vi "getStatusTime.vi"(0 "String":string, 5 "Time":dbl format="%.2f", 9 "Site":i32) -> (2 "Run":i32, 3 "RunP":i32, 4 "Down":i32, 6 "Repair":i32, 8 "Setup":i32, 10 "SetupW":i32, 13 "PM":i32, 14 "Eng":i32, 15 "Idle":i32)   [LabVIEW 2012]
panel:
  out "Repair":string
  out "PM":string
  out "Eng":string
  out "SetupW":string
  out "Setup":string
  out "Idle":string
  out "Run":string
  out "RunP":string
  out "Down":string
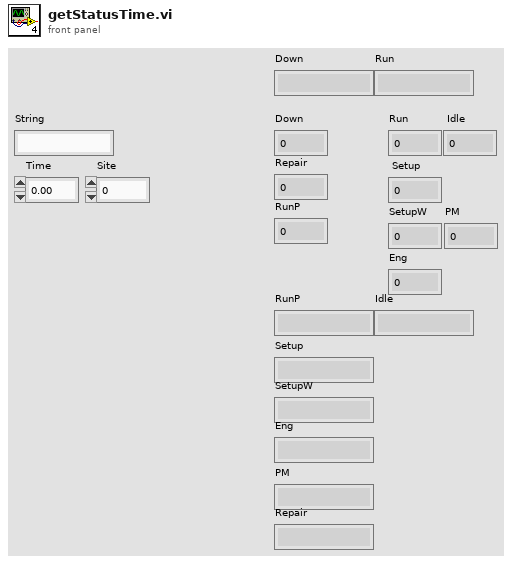
[diagram p1: front panel]
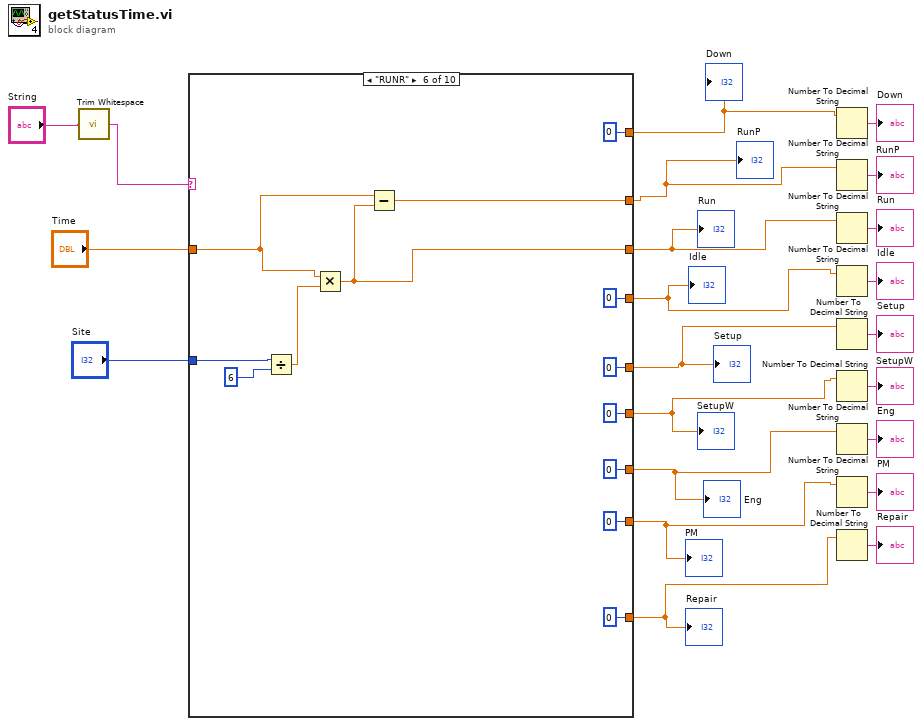
[diagram p0: block diagram]
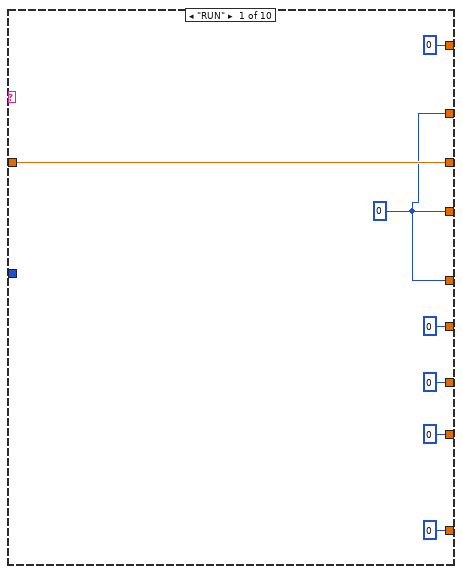
[diagram p2: hidden frame]
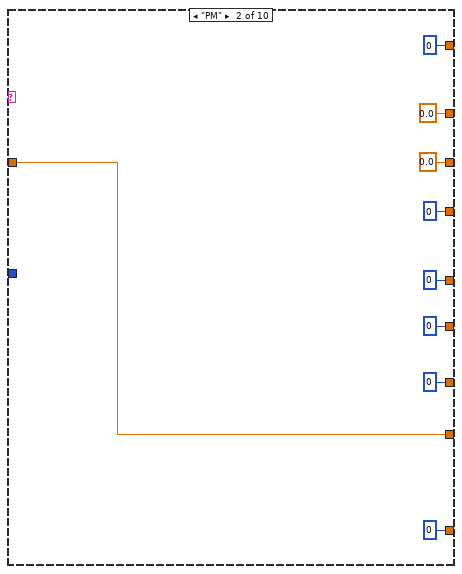
[diagram p3: hidden frame]
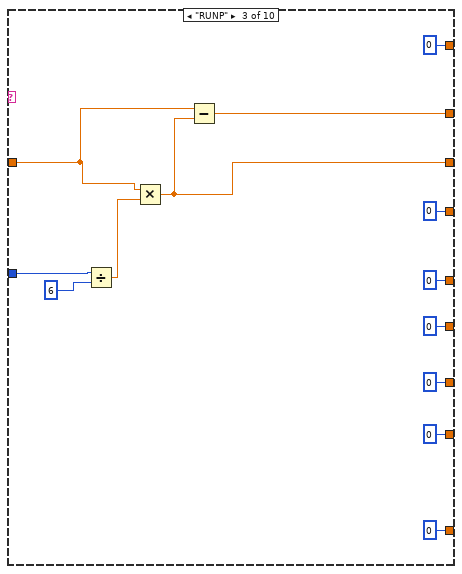
[diagram p4: hidden frame]
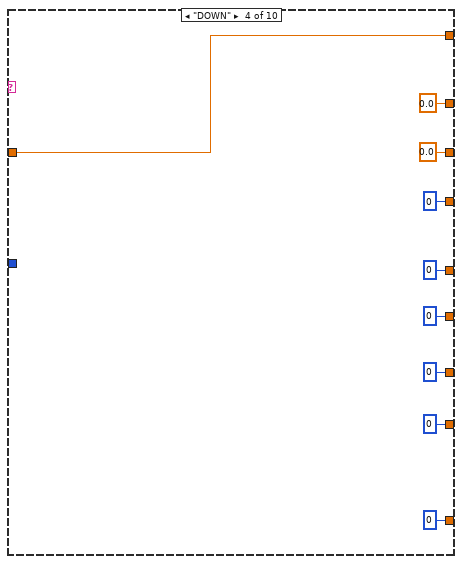
[diagram p5: hidden frame]
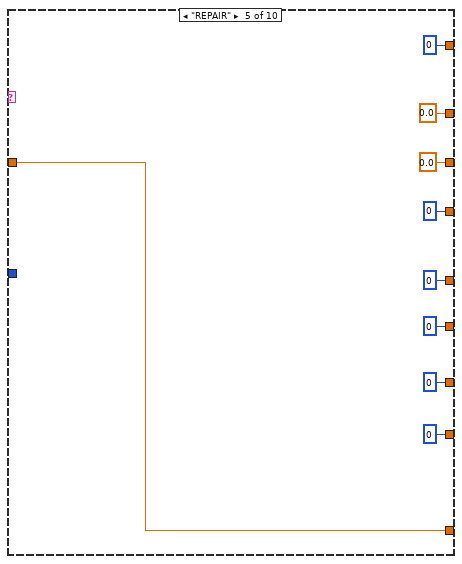
[diagram p6: hidden frame]
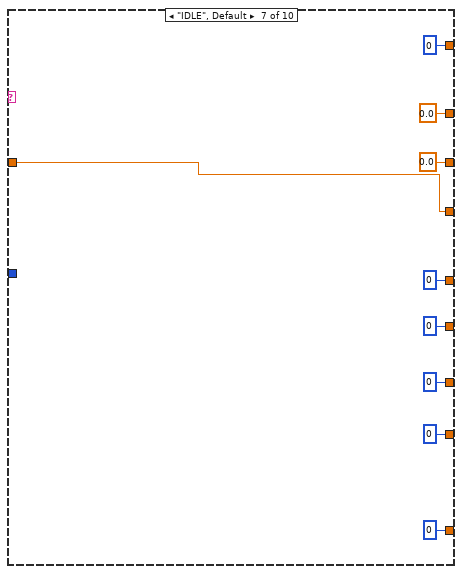
[diagram p7: hidden frame]
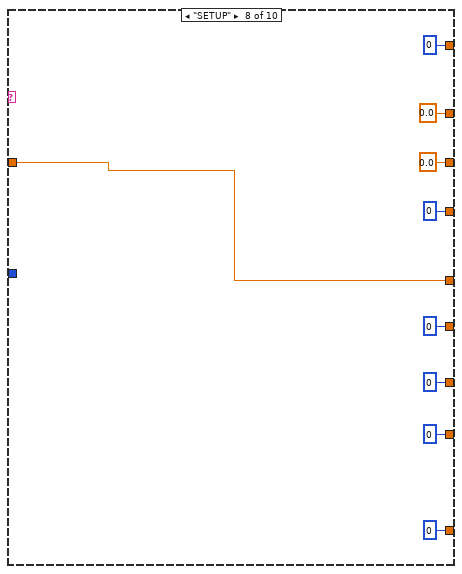
[diagram p8: hidden frame]
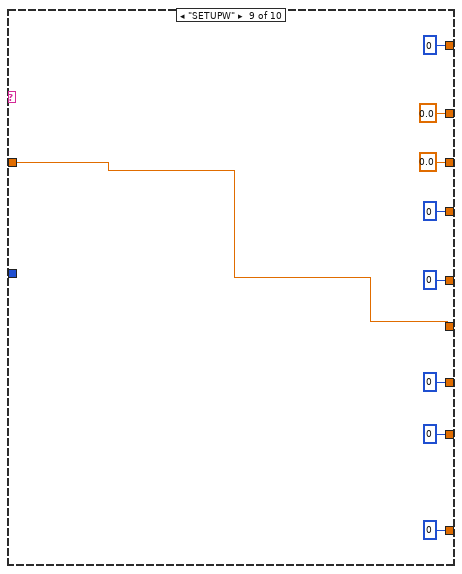
[diagram p9: hidden frame]
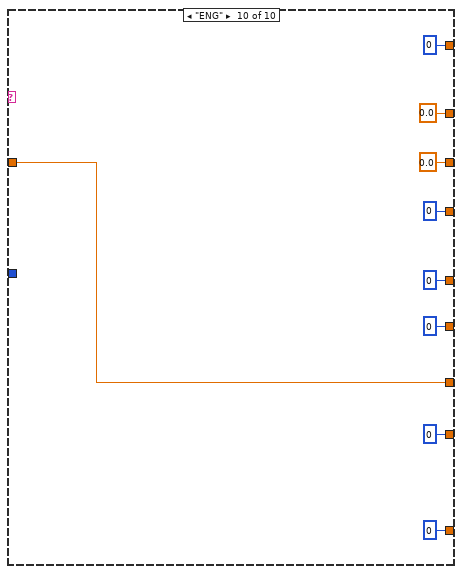
[diagram p10: hidden frame]
diagram:
  n1 = call <vilib>:"Trim Whitespace.vi"("string"="String") -> ("trimmed string"=w1:string)  [unwired: 1 in]
  n2 = case shown="\"RUNR\"" w1 {
    tunnel: "Time" -> [w29 w32 w48 w60 w69 w79 w91 w100 w106 w113]
    tunnel: [w29 0.0 ("Time") w47 0.0 ("Time") 0.0 ("Time") w78 0.0 ("Time") 0.0 ("Time") 0.0 ("Time") 0.0 ("Time")] -> w18
    tunnel: [w28 0 ("Time") 0 ("Time") 0 ("Time") 0 ("Time") 0 ("Time") w91 0 ("Time") 0 ("Time") 0 ("Time")] -> w17
    tunnel: [w28 0 ("Time") 0 ("Time") 0 ("Time") 0 ("Time") 0 ("Time") 0 w100 0 ("Time") 0 ("Time")] -> w16
    tunnel: "Site" -> [_ _ w51 _ _ w82 _ _ _ _]
    tunnel: [w28 0.0 w46 0.0 0.0 w77 0.0 0.0 0.0 0.0] -> w19
    tunnel: [0 ("Time") 0 ("Time") 0 ("Time") 0 ("Time") 0 ("Time") 0 ("Time") 0 ("Time") 0 ("Time") w106 0 ("Time")] -> w15
    tunnel: [0 ("Time") 0 ("Time") 0 ("Time") 0 ("Time") 0 ("Time") 0 ("Time") 0 ("Time") 0 ("Time") 0 ("Time") w113] -> w14
    tunnel: [0 ("Time") w32 0 ("Time") 0 ("Time") 0 ("Time") 0 ("Time") 0 ("Time") 0 ("Time") 0 ("Time") 0 ("Time")] -> w13
    tunnel: [0 ("Time") 0 ("Time") 0 ("Time") w60 0 ("Time") 0 ("Time") 0 ("Time") 0 ("Time") 0 ("Time") 0 ("Time")] -> w20
    tunnel: [0 ("Time") 0 ("Time") 0 ("Time") 0 ("Time") w69 0 ("Time") 0 ("Time") 0 ("Time") 0 ("Time") 0 ("Time")] -> w12
    frame "RUN" {
      w28 = 0
    }
    frame "PM" {
    }
    frame "RUNP" {
      n3 = Divide(x=w51, y=6) -> (x/y=w49:dbl)
      n4 = Multiply(x=w48, y=w49) -> (x*y=w47:dbl)
      n5 = Subtract(x=w48, y=w47) -> (x-y=w46:dbl)
    }
    frame "DOWN" {
    }
    frame "REPAIR" {
    }
    frame "RUNR" {
      n6 = Divide(x=w82, y=6) -> (x/y=w80:dbl)
      n7 = Multiply(x=w79, y=w80) -> (x*y=w78:dbl)
      n8 = Subtract(x=w79, y=w78) -> (x-y=w77:dbl)
    }
    frame "IDLE", Default {
    }
    frame "SETUP" {
    }
    frame "SETUPW" {
    }
    frame "ENG" {
    }
  }
  "Run" <- w18
  "Idle" <- w17
  "Setup" <- w16
  "SetupW" <- w15
  "Eng" <- w14
  "PM" <- w13
  "Down" <- w20
  "Repair" <- w12
  "RunP" <- w19
  n9 = Number To Decimal String(number=w20) -> (decimal integer string=→"Down":string)  [unwired: 1 in]
  n10 = Number To Decimal String(number=w19) -> (decimal integer string=→"RunP":string)  [unwired: 1 in]
  n11 = Number To Decimal String(number=w18) -> (decimal integer string=→"Run":string)  [unwired: 1 in]
  n12 = Number To Decimal String(number=w17) -> (decimal integer string=→"Idle":string)  [unwired: 1 in]
  n13 = Number To Decimal String(number=w16) -> (decimal integer string=→"Setup":string)  [unwired: 1 in]
  n14 = Number To Decimal String(number=w15) -> (decimal integer string=→"SetupW":string)  [unwired: 1 in]
  n15 = Number To Decimal String(number=w14) -> (decimal integer string=→"Eng":string)  [unwired: 1 in]
  n16 = Number To Decimal String(number=w13) -> (decimal integer string=→"PM":string)  [unwired: 1 in]
  n17 = Number To Decimal String(number=w12) -> (decimal integer string=→"Repair":string)  [unwired: 1 in]
